vi "SavePointables.vi"(10 "error in (no error)":errorcluster, 11 "Leap Pointables":refnum<k24>) -> (2 "error out":errorcluster, 3 "Pointables":T1[](array[typedef]))   [LabVIEW 2010, in "lvleap.lvlib"]
uses:
  lvleap.lvlib
  Controls/Pointable.ctl
  Controls/Pointable Type.ctl
  Controls/Vector.ctl
  Controls/Pointable Zone.ctl
  C:/Users/mraj/Desktop/src/Libs/LeapCSharp.NET3.5.dll
  Libs/LeapCSharp.NET3.5.dll
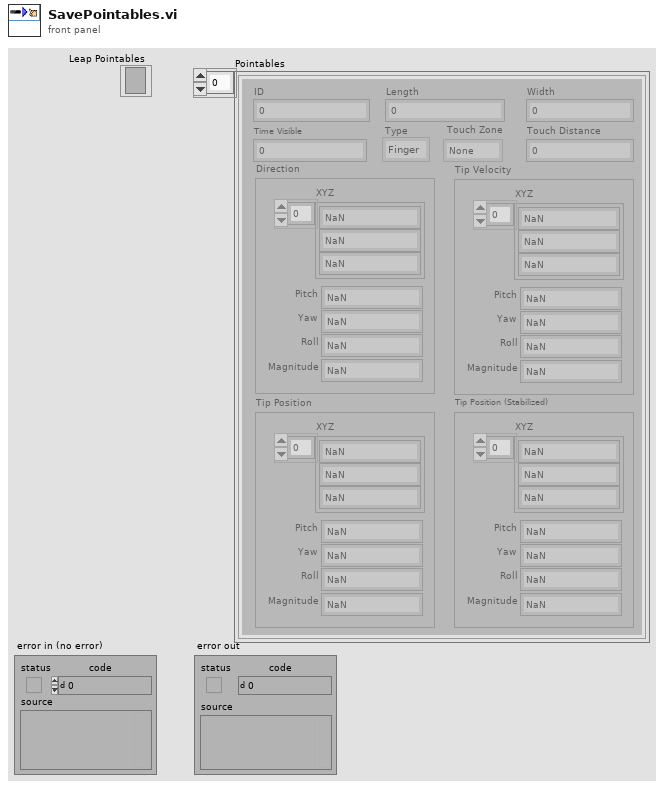
[diagram p1: front panel]
types:
  T1 = typedef "lvleap.lvlib/Pointable.ctl" = cluster{"ID":i32, "Length":dbl, "Width":dbl, "Time Visible":dbl, "Type":T2, "Direction":T3, "Tip Velocity":T3, "Tip Position":T3, "Tip Position (Stabilized)":T3, "Touch Zone":T4, "Touch Distance":dbl}
  T2 = typedef "lvleap.lvlib/Pointable Type.ctl" = enum16{"Finger", "Tool"}
  T3 = typedef "lvleap.lvlib/Vector.ctl" = cluster{"Pitch":sgl, "Yaw":sgl, "Roll":sgl, "Magnitude":sgl, "XYZ":sgl[]}
  T4 = typedef "lvleap.lvlib/Pointable Zone.ctl" = enum16{"None", "Hovering", "Touching"}
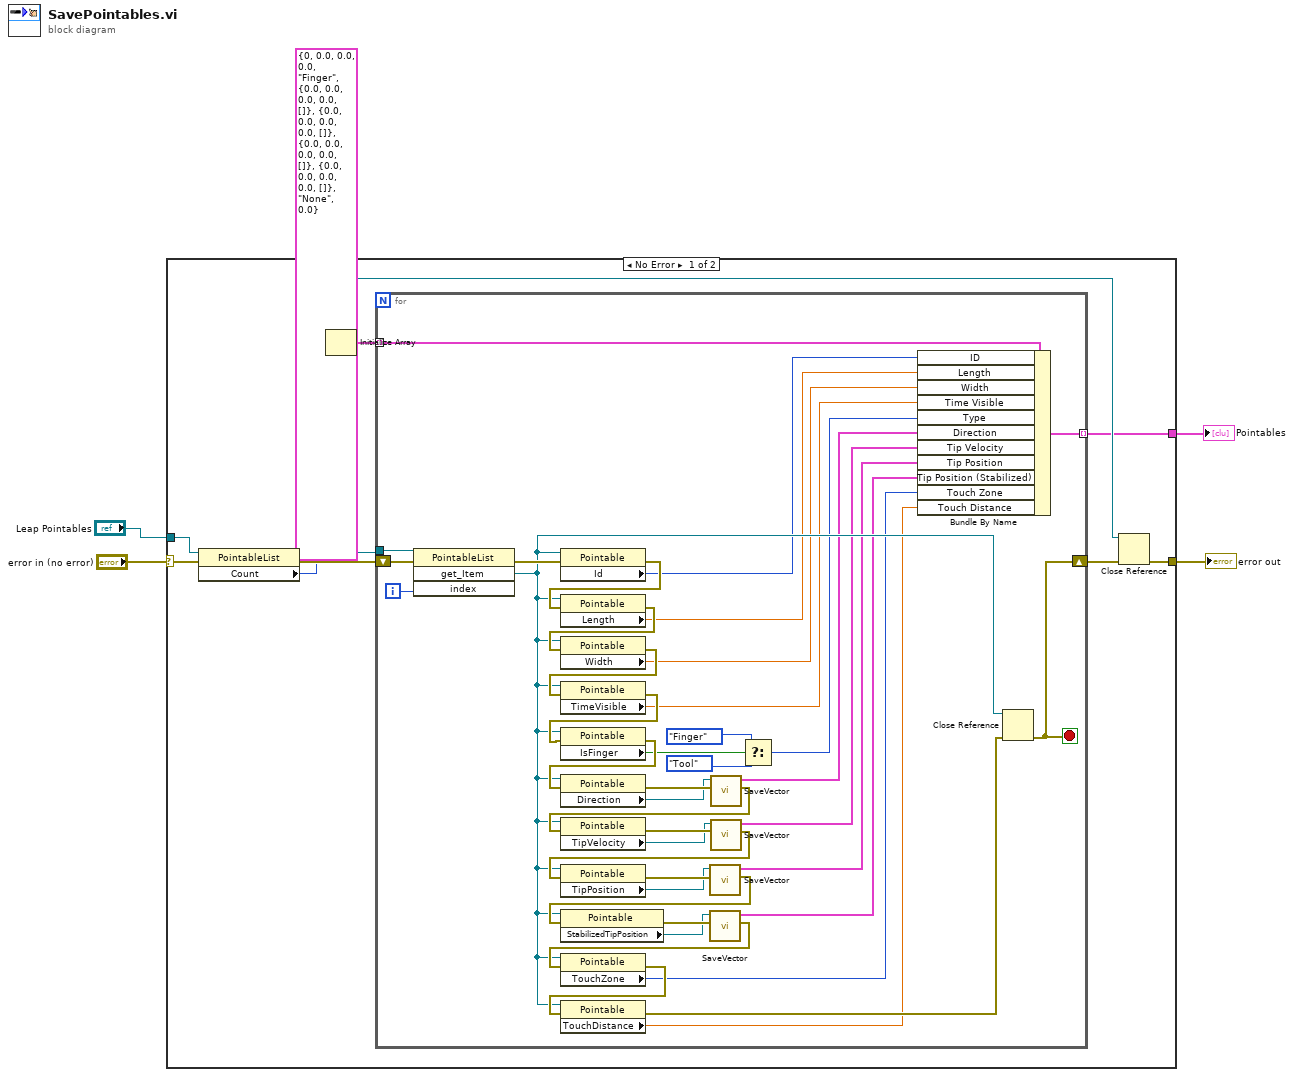
[diagram p0: block diagram]
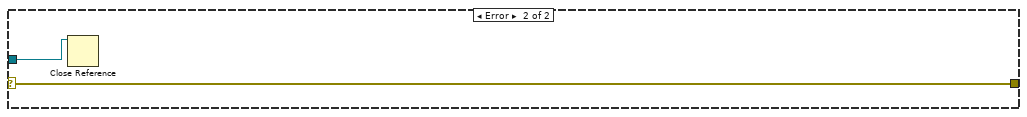
[diagram p2: hidden frame]
diagram:
  n1 = case shown="No Error" "error in (no error)" {
    selector: "error in (no error)" -> [w8 w57]
    tunnel: [w12 _] -> w2
    tunnel: "Leap Pointables" -> [w9 w56]
    tunnel: [w6 w57] -> w3
    frame No Error {
      n2 = property class="PointableList"(reference=w9, error in=w8) -> (reference out=w13:refnum<k24>, error out=w14:errorcluster, "Count"=w10:i32)
      n3 = Initialize Array(T1 {"ID"=0, "Length"=0.0, "Width"=0.0, "Time Visible"=0.0, "Type"=enum."Finger", "Direction"={"Pitch"=0.0, "Yaw"=0.0, "Roll"=0.0, "Magnitude"=0.0, "XYZ"=[]}, "Tip Velocity"={"Pitch"=0.0, "Yaw"=0.0, "Roll"=0.0, "Magnitude"=0.0, "XYZ"=[]}, "Tip Position"={"Pitch"=0.0, "Yaw"=0.0, "Roll"=0.0, "Magnitude"=0.0, "XYZ"=[]}, "Tip Position (Stabilized)"={"Pitch"=0.0, "Yaw"=0.0, "Roll"=0.0, "Magnitude"=0.0, "XYZ"=[]}, "Touch Zone"=enum."None", "Touch Distance"=0.0} ("Finger"), w10) -> (w11:T1[])
      n4 = for {
        tunnel: w13 -> [w41]
        tunnel: w11 -> [w39] mode=indexing
        tunnel: [w38] -> w12 mode=indexing
        shift-right: [w29] -> w7
        shift-left: w14 -> [w42]
        i -> [w40]
        stop <- w29 stop-if-true
        n5 = invoke class="PointableList" method="get_Item"(reference=w41, error in=w42, "index"=w40) -> (error out=w55:errorcluster, "get_Item"=w44:refnum<k24>)  [unwired: 1 in, 2 out]
        n6 = property class="Pointable"(reference=w44, error in=w55) -> (error out=w45:errorcluster, "Id"=w30:i32)  [unwired: 1 out]
        n7 = property class="Pointable"(reference=w44, error in=w45) -> (error out=w46:errorcluster, "Length"=w31:sgl)  [unwired: 1 out]
        n8 = property class="Pointable"(reference=w44, error in=w46) -> (error out=w47:errorcluster, "Width"=w32:sgl)  [unwired: 1 out]
        n9 = property class="Pointable"(reference=w44, error in=w47) -> (error out=w48:errorcluster, "TimeVisible"=w22:sgl)  [unwired: 1 out]
        n10 = property class="Pointable"(reference=w44, error in=w48) -> (error out=w49:errorcluster, "IsFinger"=w26:bool)  [unwired: 1 out]
        n11 = property class="Pointable"(reference=w44, error in=w49) -> (error out=w43:errorcluster, "Direction"=w33:refnum<k24>)  [unwired: 1 out]
        n12 = call "SaveVector.vi"("error in (no error)"=w43, "Leap Vector"=w33) -> ("error out"=w50:errorcluster, "Vector"=w20:T3)  [unwired: 8 in]
        n13 = property class="Pointable"(reference=w44, error in=w50) -> (error out=w35:errorcluster, "TipVelocity"=w34:refnum<k24>)  [unwired: 1 out]
        n14 = call "SaveVector.vi"("error in (no error)"=w35, "Leap Vector"=w34) -> ("error out"=w51:errorcluster, "Vector"=w19:T3)  [unwired: 8 in]
        n15 = property class="Pointable"(reference=w44, error in=w51) -> (error out=w37:errorcluster, "TipPosition"=w36:refnum<k24>)  [unwired: 1 out]
        n16 = call "SaveVector.vi"("error in (no error)"=w37, "Leap Vector"=w36) -> ("error out"=w52:errorcluster, "Vector"=w18:T3)  [unwired: 8 in]
        n17 = property class="Pointable"(reference=w44, error in=w52) -> (error out=w28:errorcluster, "StabilizedTipPosition"=w27:refnum<k24>)  [unwired: 1 out]
        n18 = call "SaveVector.vi"("error in (no error)"=w28, "Leap Vector"=w27) -> ("error out"=w53:errorcluster, "Vector"=w17:T3)  [unwired: 8 in]
        n19 = property class="Pointable"(reference=w44, error in=w53) -> (error out=w54:errorcluster, "TouchZone"=w16:i32)  [unwired: 1 out]
        n20 = property class="Pointable"(reference=w44, error in=w54) -> (error out=w23:errorcluster, "TouchDistance"=w15:sgl)  [unwired: 1 out]
        n21 = Select(t=Pointable_Type."Finger" ("pointable type"), s=w26, f=Pointable_Type."Tool" ("pointable type")) -> (s? t:f=w21:T2)
        n22 = Bundle By Name(cluster=w39, "ID"=w30, "Length"=w31, "Width"=w32, "Time Visible"=w22, "Type"=w21, "Direction"=w20, "Tip Velocity"=w19, "Tip Position"=w18, "Tip Position (Stabilized)"=w17, "Touch Zone"=w16, "Touch Distance"=w15) -> (w38:T1)
        n23 = Close Reference(reference=w44, error in (no error)=w23) -> (error out=w29:errorcluster)
      }
      n24 = Close Reference(reference=w13, error in (no error)=w7) -> (error out=w6:errorcluster)
    }
    frame Error {
      n25 = Close Reference(reference=w56) -> ()  [unwired: 1 in, 1 out]
    }
  }
  "Pointables" <- w2
  "error out" <- w3
